vi "QuadBot Initialise.vi"(8 "error in (no error)":errorcluster, 10 "Start Position":enum16{"Sitting", "Standing", "None"}(ring), 11 "Cluster":cluster{"Ctl Refnum":refnum<vi>}) -> (0 "error out":errorcluster, 3 "Cluster 2":cluster{"Ctl Refnum 2":refnum<vi>})   [LabVIEW 2015]
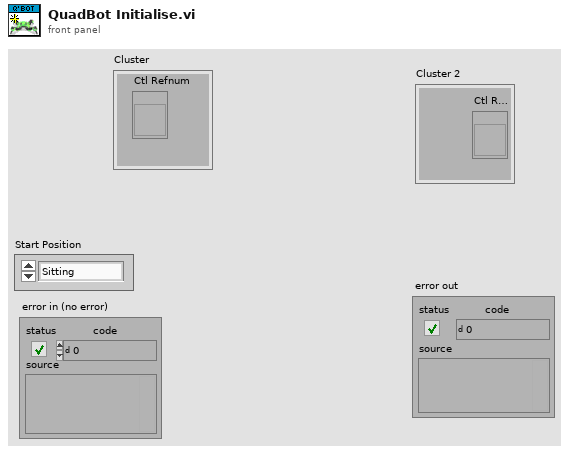
[diagram p1: front panel]
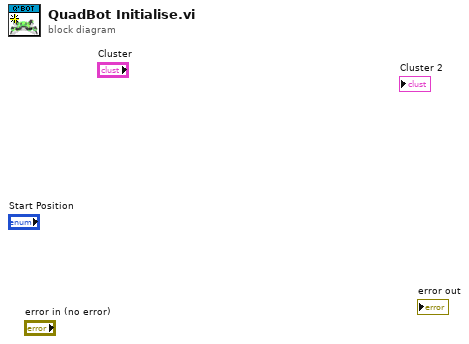
[diagram p0: block diagram]
diagram:
